vi "get_Trajectory.vi"(8 "error in (no error)":errorcluster, 11 "ScanModeDL090923Scaffold in":refnum<class "ImagingModeDL090923Scaffold.lvclass">) -> (0 "error out":errorcluster, 1 "Trajectory adapter":refnum<class "GenericAdapter.lvclass">, 2 "Trajectory":refnum<class "GenericTrajectory.lvclass">, 3 "ScanModeDL090923Scaffold out":refnum<class "ImagingModeDL090923Scaffold.lvclass">, 4 "specification":T1, 5 "to-ImageAssembler adapter":refnum<class "GenericAdapter.lvclass">, 6 "adapter path":path, 7 "Trajectory-to-ImageAssembler adapter path":path)   [LabVIEW 2010, in "ImagingModeDL090923Scaffold.lvclass"]
uses:
  ImagingModeDL090923Scaffold.lvclass
  Trajectory/GenericTrajectory/GenericTrajectory/GenericTrajectory.lvclass
  Adapter/GenericAdapter/GenericAdapter/GenericAdapter.lvclass
  common/clusters/plugin_specification.ctl
  ImagingModeDL090923Scaffold.lvclass/ImagingModeDL090923Scaffold.ctl
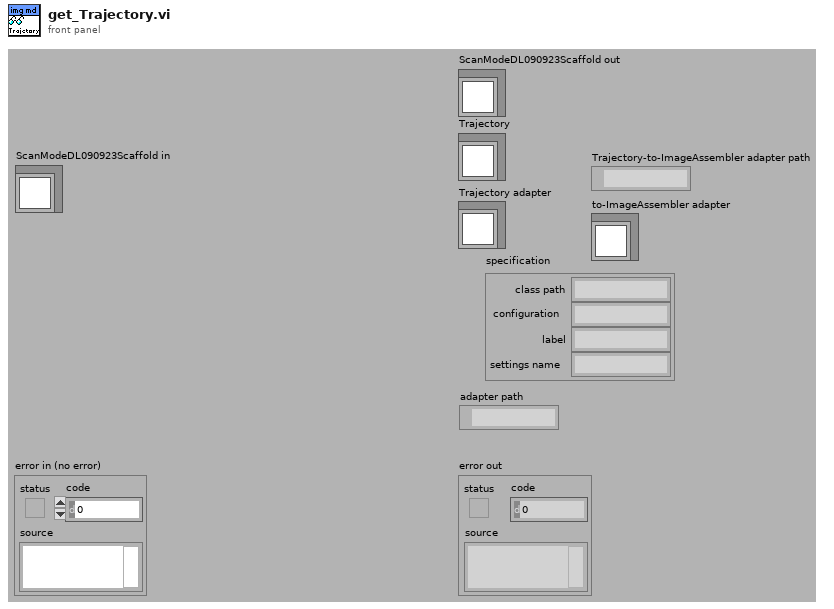
[diagram p1: front panel]
types:
  T1 = typedef "plugin_specification.ctl" = cluster{"class path":string, "configuration":string, "label":string, "settings name":string}
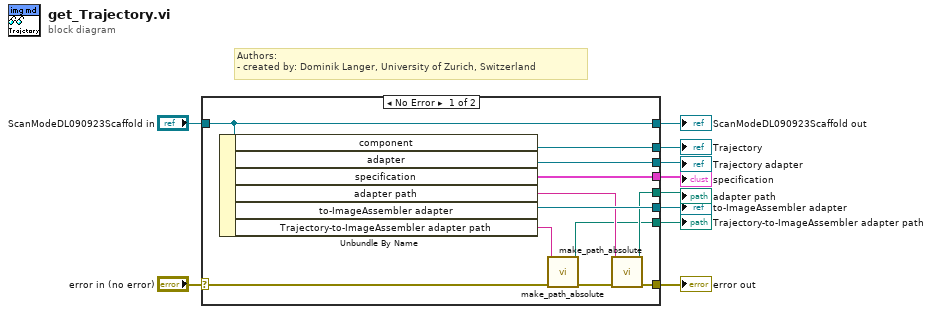
[diagram p0: block diagram]
diagram:
  # "Authors: \n- created by: Dominik Langer, University of Zurich, Switzerland"
  n1 = case shown="No Error" "error in (no error)" {
    selector: "error in (no error)" -> [w12 w23]
    tunnel: [w15 w23] -> w9
    tunnel: [w22 w24] -> w7
    tunnel: "ScanModeDL090923Scaffold in" -> [w22 w24]
    tunnel: [w21 _] -> w6
    tunnel: [w20 _] -> w5
    tunnel: [w19 _] -> w4
    tunnel: [w16 _] -> w3
    tunnel: [w18 _] -> w2
    tunnel: [w13 _] -> w1
    frame No Error {
      n2 = Unbundle By Name(w22) -> ("component"=w21:refnum<class "GenericTrajectory.lvclass">, "adapter"=w20:refnum<class "GenericAdapter.lvclass">, "specification"=w19:T1, "adapter path"=w17:string, "to-ImageAssembler adapter"=w18:refnum<class "GenericAdapter.lvclass">, "Trajectory-to-ImageAssembler adapter path"=w14:string)
      n3 = call "make_path_absolute.vi"("error in (no error)"=w12, "relative path"=w14) -> ("error out"=w11:errorcluster, "absolute path"=w13:path)  [unwired: 8 in]
      n4 = call "make_path_absolute.vi"("error in (no error)"=w11, "relative path"=w17) -> ("error out"=w15:errorcluster, "absolute path"=w16:path)  [unwired: 8 in]
    }
    frame Error {
    }
  }
  "error out" <- w9
  "ScanModeDL090923Scaffold out" <- w7
  "Trajectory" <- w6
  "Trajectory adapter" <- w5
  "specification" <- w4
  "adapter path" <- w3
  "to-ImageAssembler adapter" <- w2
  "Trajectory-to-ImageAssembler adapter path" <- w1
